vi "Periodic Tasks.vi"(8 "error in":errorcluster) -> ()   [LabVIEW 2023]
doc: "This VI runs in parallel to other tasks. It can contain as many user-defined periodic loops as you need. These can carry out PID or other sorts of timed response."
uses:
  Global odometry.vi
  <vilib>/Rock Robotics/WPI/ThirdParty/Phoenix-LabVIEW/CANCoder/Get/CTRE_Phoenix_CANcoder_GetSensorData.vi
  Global INIT.vi
panel:
  in  "Tab Control":enum32{"Page 1", "Page 2", "Page 3"}(tab)
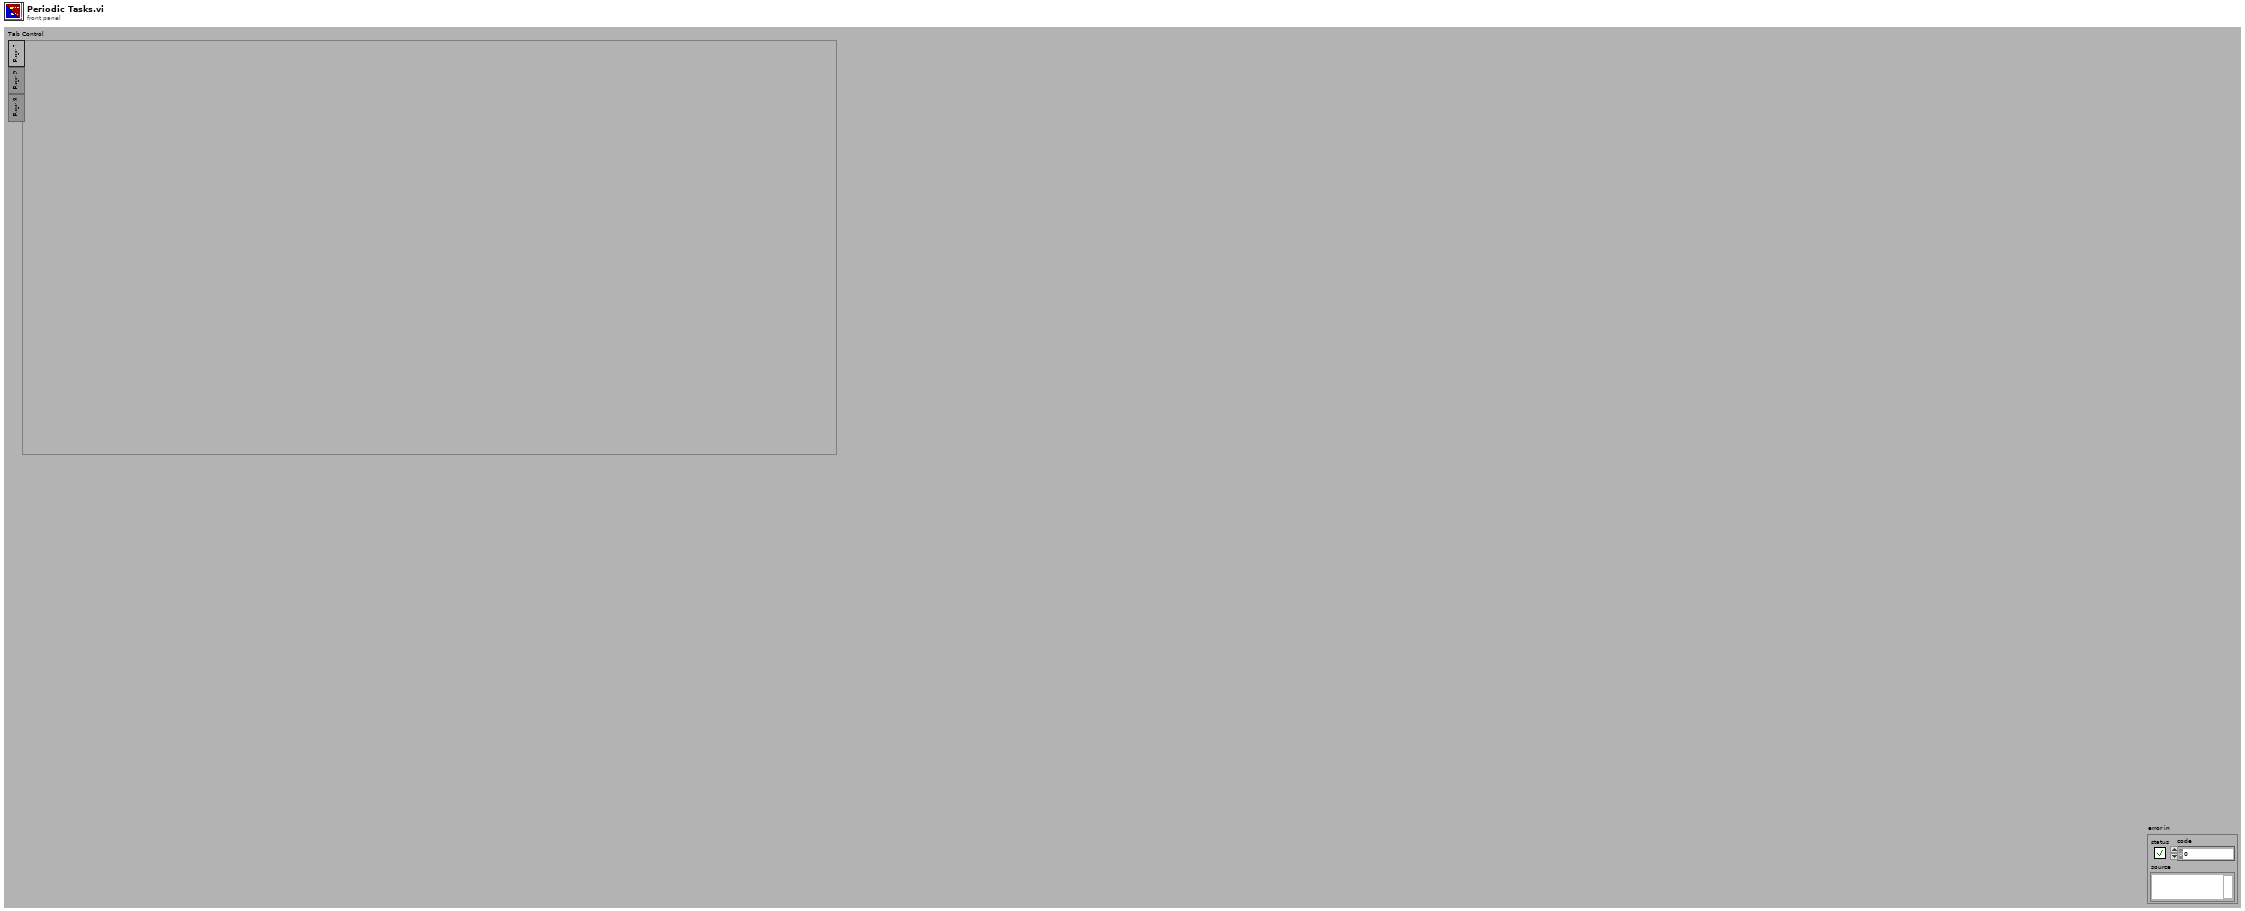
[diagram p1: front panel]
types:
  T1 = typedef "WPI_MotorControlDeviceRef.ctl" = cluster{"DeviceStatus":errorcluster, "Type":T2, "PWM":cluster{"PWM Channel":T3, "DeadBand":T4}, "CAN":cluster{"Device Number":u8, "SetOutput VI Ref":variant, "GetOutput VI Ref":variant, "Enable VI Ref":variant, "Disable VI Ref":variant, "Data":variant}, "Invert":bool, "DIO PWM":cluster{"PWM \"Enable\" Channel":T3, "DIOChannel":T5, "PWM Rate":dbl}}
  T2 = typedef "WPI_MotorControlType.ctl" = enum16{"PWM", "CAN", "DIO PWM"}
  T3 = typedef "FPGA_DIOPWMChannel.ctl" = enum8{"PWM 0", "PWM 1", "PWM 2", "PWM 3", "PWM 4", "PWM 5", "PWM 6", "PWM 7", "PWM 8", "PWM 9", "PWM MXP 0", "PWM MXP 1", "PWM MXP 2", "PWM MXP 3", "PWM MXP 4", "PWM MXP 5", "PWM MXP 6", "PWM MXP 7", "PWM MXP 8", "PWM MXP 9", "Invalid"}
  T4 = typedef "WPI_PWMDeadband.ctl" = cluster{"Name":string, "maxPositivePwm":i32, "minPositivePwm":i32, "centerPwm":i32, "maxNegativePwm":i32, "minNegativePwm":i32, "angularRange":u16}
  T5 = typedef "FPGA_DIOChannel.ctl" = enum8{"DIO 0", "DIO 1", "DIO 2", "DIO 3", "DIO 4", "DIO 5", "DIO 6", "DIO 7", "DIO 8", "DIO 9", "DIO MXP 0", "DIO MXP 1", "DIO MXP 2", "DIO MXP 3", "DIO MXP 4", "DIO MXP 5", "DIO MXP 6", "DIO MXP 7", "DIO MXP 8", "DIO MXP 9", "DIO MXP 10", "DIO MXP 11", "DIO MXP 12", "DIO MXP 13", "DIO MXP 14", "DIO MXP 15", "SPI Port CS1", "SPI Port CS2", "SPI Port CS3", "SPI Port MISO", "SPI Port MOSI", "Invalid"}
  T6 = typedef "CTRE_Phoenix_CANcoder_DeviceRef.ctl" = cluster{"DeviceStatus":errorcluster, "Device Number":u8, "Handle":u64, "UsageFrame":u32, "Library Path":path}
  T7 = cluster{"Yaw":dbl, "Roll":dbl, "Pitch":dbl, "Heading":dbl, "Fused Heading":dbl}
  T8 = typedef "ctrl DRIVING FRAME selector.ctl" = enum16{"ROBO-centric", "FLD-centric"}
  T9 = typedef "ctrl FRONT FACE selector.ctl" = enum16{"intake side", "shooter side"}
  T10 = typedef "WPI_DriverStationAllianceInfo.ctl" = enum16{"Red", "Blue", "Invalid"}
  T11 = typedef "ctrl swerve module.ctl" = cluster{"descr":string, "V":dbl, "POS":dbl, "target":dbl, "ABS":dbl, "from pivot to module":cluster{"R":dbl, "theta (deg)":dbl, "theta spin (deg)":dbl}, "coord wrt geom CTR":cluster{"X":dbl, "Y":dbl}, "corner wt (lbm)":dbl}
  T12 = typedef "ctrl solenoid.ctl" = cluster{"description":string, "Installed?":bool, "refnum name":string, "coils":enum16{"Single", "Double"}, "forward channel":T13, "reverse channel":T13, "initial value":T14}
  T13 = typedef "WPI_SolenoidChannel.ctl" = enum8{"Solenoid 0", "Solenoid 1", "Solenoid 2", "Solenoid 3", "Solenoid 4", "Solenoid 5", "Solenoid 6", "Solenoid 7", "Solenoid 8", "Solenoid 9", "Solenoid 10", "Solenoid 11", "Solenoid 12", "Solenoid 13", "Solenoid 14", "Solenoid 15", "Invalid"}
  T14 = typedef "WPI_SolenoidValue.ctl" = enum16{"Off", "On", "Forward", "Reverse"}
  T15 = typedef "ctrl arm motor.ctl" = cluster{" motor":T16, "limit polarities":T19}
  T16 = typedef "ctrl swerve motor.ctl" = cluster{"description":string, "Installed?":bool, "CAN ID":u8, "refnum name":string, "Invert":bool, "Idle Mode":T17, "Current limiting":T18}
  T17 = typedef "Spark MAX Idle Mode.ctl" = enum16{"Coast", "Brake"}
  T18 = typedef "ctrl Spark MAX current limiting.ctl" = cluster{"Linearized Limit Enabled (F)":bool, "Free Speed Current Limit (20A)":dbl, "Primay Current Limit (80A)":dbl, "Linear Limit RPM (0)":u32}
  T19 = typedef "ctrl limit polarity.ctl" = cluster{"Forward limit":T20, "Reverse limit":T20}
  T20 = typedef "Spark MAX Limit Switch Polarity.ctl" = enum16{"Normally Open", "Normally Closed"}
  T21 = cluster{"LEFT ARM":cluster{"VBus%":dbl, "LOCK?":bool, "LOCKED":bool}, "RIGHT ARM":cluster{"VBus%":dbl, "LOCK?":bool, "LOCKED":bool}}
  T22 = cluster{"VBus%":dbl, "LOCK?":bool, "LOCKED":bool}
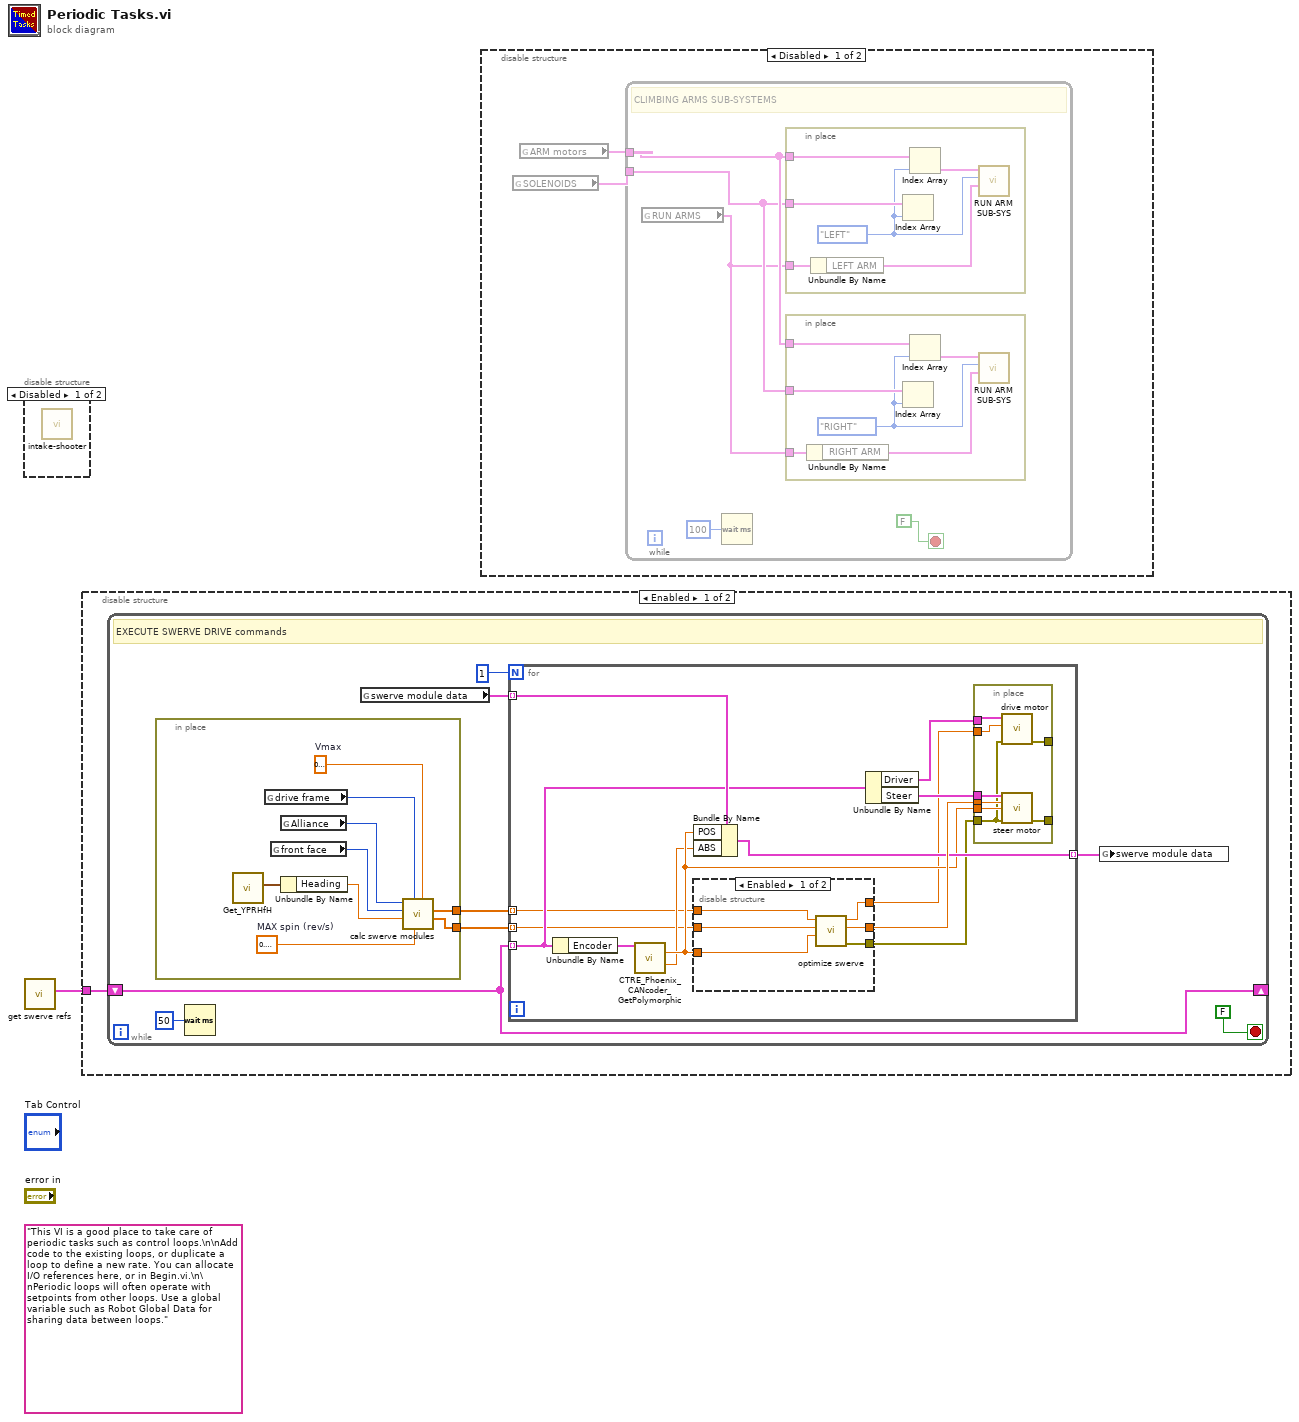
[diagram p0: block diagram]
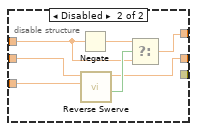
[diagram p4: hidden frame]
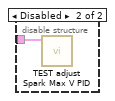
[diagram p5: hidden frame]
diagram:
  (unwired) "This VI is a good place to take care of periodic tasks such as control loops.\n\nAdd code to the existing loops, or duplicate a loop to define a new rate. You can allocate I/O references here, or in Begin.vi.\n\nPeriodic loops will often operate with setpoints from other loops. Use a global variable such as Robot Global Data for sharing data between loops."
  n1 = disable-structure shown="Disabled" {
    frame Disabled {
      n2 = call "intake-shooter.vi"() -> ()  [unwired: 12 in]
    }
    frame Enabled {
    }
  }
  n3 = call "get swerve refs.vi"() -> ("Swerve refs"=w1:cluster{"Driver":T1, "Steer":T1, "Encoder":T6}[])  [unwired: 10 in, 1 out]
  n4 = disable-structure shown="Enabled" {
    disable-tunnel: w1 -> [w2 w54]
    frame Enabled {
      n5 = while {
        shift-right: [w8] -> _
        shift-left: w2 -> [w8]
        stop <- FALSE stop-if-true
        # "EXECUTE SWERVE DRIVE commands"
        n6 = in-place {
          in-place-border: [w17] -> w4
          in-place-border: [w16] -> w3
          w18 = 0.7000000000000001  # MAX spin (rev/s)
          w19 = 0.9999999999999992  # Vmax
          n7 = call <vilib>:"Get_YPRHfH.vi"() -> ("YRPHfH"=w15:T7)  [unwired: 11 in]
          n8 = global read "Global odometry.vi" "drive frame"() -> (w13:T8)
          n9 = global read "Global odometry.vi" "front face"() -> (w11:T9)
          n10 = global read "Global odometry.vi" "Alliance"() -> (w12:T10)
          n11 = Unbundle By Name(w15) -> ("Heading"=w14:dbl)
          n12 = call "calc swerve modules.vi"("Vmax"=w19, "MAX spin (rev/s)"=w18, "drive frame"=w13, "HDG (deg)"=w14, "front face"=w11, "Alliance"=w12) -> ("angle"=w16:dbl[], "speed norm"=w17:dbl[])  [unwired: 4 in]
        }
        n13 = Wait (ms)(milliseconds to wait=u32 50) -> ()  [unwired: 1 out]
        n14 = global read "Global odometry.vi" "swerve module data"() -> (w6:T11[])
        n15 = for {
          N: 1 -> [_]
          tunnel: w8 -> [w24] mode=indexing
          tunnel: w6 -> [w30] mode=indexing
          tunnel: [w29] -> w5 mode=indexing
          tunnel: w4 -> [w21] mode=indexing
          tunnel: w3 -> [w20] mode=indexing
          n16 = Unbundle By Name(w24) -> ("Encoder"=w23:T6)
          n17 = call-poly <vilib>:"CTRE_Phoenix_CANcoder_GetPolymorphic.vi"("CTRE_CANcoder_DeviceRef"=w23) -> ("Position"=w28:dbl, "Absolute Position"=w27:dbl)  [unwired: 10 in, 3 out]
          n18 = Bundle By Name(cluster=w30, "POS"=w28, "ABS"=w27) -> (w29:T11)
          n19 = disable-structure shown="Enabled" {
            disable-tunnel: [w38 w41] -> w32
            disable-tunnel: w21 -> [w37 w43]
            disable-tunnel: w20 -> [w33 w40]
            disable-tunnel: w28 -> [w36 w39]
            disable-tunnel: [w35 w44] -> w25
            disable-tunnel: [w34 _] -> w22
            frame Enabled {
              n20 = call "optimize swerve.vi"("current angle (deg)"=w36, "target angle (deg)"=w33, "velocity"=w37) -> ("error out"=w34:errorcluster, "steer angle (deg)"=w38:dbl, "velocity"=w35:dbl)  [unwired: 5 in, 1 out]
            }
            frame Disabled {
              n21 = Negate(x=w43) -> (-x=w42:dbl)
              n22 = call "Reverse Swerve.vi"("POSold"=w39, "Joystick Value"=w40) -> ("Reversed"=w45:bool, "POSnew"=w41:dbl)  [unwired: 7 in, 1 out]
              n23 = Select(t=w42, s=w45, f=w43) -> (s? t:f=w44:dbl)
            }
          }
          n24 = Unbundle By Name(w24) -> ("Driver"=w26:T1, "Steer"=w31:T1)
          n25 = in-place {
            in-place-border: w32 -> [w53]
            in-place-border: w31 -> [w52]
            in-place-border: w28 -> [w51]
            in-place-border: w26 -> [w50]
            in-place-border: w25 -> [w49]
            in-place-border: w22 -> [w48]
            in-place-border: [w47] -> _
            in-place-border: [w46] -> _
            n26 = call "drive motor.vi"("error in (no error)"=w48, "velocity"=w49, "Driver"=w50) -> ("error out"=w47:errorcluster)  [unwired: 8 in]
            n27 = call "steer motor.vi"("MotorControlDevRef"=w52, "target"=w53, "encoder"=w51, "error in (no error)"=w48) -> ("error out"=w46:errorcluster)  [unwired: 11 in]
          }
        }
        n28 = global write "Global odometry.vi" "swerve module data"(w5) -> ()
      }
    }
    frame Disabled {
      n29 = call "TEST adjust Spark Max V PID.vi"("Swerve refs"=w54) -> ()  [unwired: 11 in]
    }
  }
  n30 = disable-structure shown="Disabled" {
    frame Disabled {
      n31 = global read "Global INIT.vi" "SOLENOIDS"() -> (w56:T12[])
      n32 = global read "Global INIT.vi" "ARM motors"() -> (w55:T15[])
      n33 = while {
        tunnel: w56 -> [w58]
        tunnel: w55 -> [w59]
        stop <- FALSE stop-if-true
        # "CLIMBING ARMS SUB-SYSTEMS"
        n34 = global read "Global odometry.vi" "RUN ARMS"() -> (w57:T21)
        n35 = Wait (ms)(milliseconds to wait=u32 100) -> ()  [unwired: 1 out]
        n36 = in-place {
          in-place-border: w59 -> [w72]
          in-place-border: w58 -> [w70]
          in-place-border: w57 -> [w69]
          w68 = enum16{"LEFT", "RIGHT"}."LEFT" ("SIDE")
          n37 = Unbundle By Name(w69) -> ("LEFT ARM"=w73:T22)
          n38 = Index Array(array=w70, index=w68) -> ()  [unwired: 1 out]
          n39 = Index Array(array=w72, index=w68) -> (element=w71:T15)
          n40 = call "RUN ARM SUB-SYS.vi"("ARM"=w73, "SIDE"=w68, "ARM motor"=w71) -> ()  [unwired: 9 in]
        }
        n41 = in-place {
          in-place-border: w59 -> [w66]
          in-place-border: w58 -> [w64]
          in-place-border: w57 -> [w63]
          w62 = enum16{"LEFT", "RIGHT"}."RIGHT" ("SIDE")
          n42 = Unbundle By Name(w63) -> ("RIGHT ARM"=w67:T22)
          n43 = Index Array(array=w64, index=w62) -> ()  [unwired: 1 out]
          n44 = Index Array(array=w66, index=w62) -> (element=w65:T15)
          n45 = call "RUN ARM SUB-SYS.vi"("ARM"=w67, "SIDE"=w62, "ARM motor"=w65) -> ()  [unwired: 9 in]
        }
      }
    }
    frame Enabled {
    }
  }
